vi "Main_17B.vi"() -> ()   [LabVIEW 2024]
uses:
  MAP_Registers.ctl
  ENUM_Instructions.ctl
  <vilib>/Utility/error.llb/Trim Whitespace One-Sided.vi
  Utility/Universal Utility/TypeDefs_Utility/Cluster_Row-Column.ctl
  ENUM_Combo Select.ctl
panel:
  out "Program itteration":i32
  out "A Itteration":i32
  out "Answer":i32
  out "Register start":T1
  out "Output":i32[](array[numeric])
  out "Register end":T1
  in  "Select Data":enum32{"Example", "Puzzle"}(tab)
  in  "Example":string="Register A: 2024\nRegister B: 0\nRegister C: 0\n\nProgram: 0,3,5,4,3,0"
  in  "Puzzle":string="Register A: 60589763\nRegister B: 0\nRegister C: 0\n\nProgram: 2,4,1,5,7,5,1,6,4,1,5,5,0,3,3,0"
  out "Program":i32[](array[numeric])
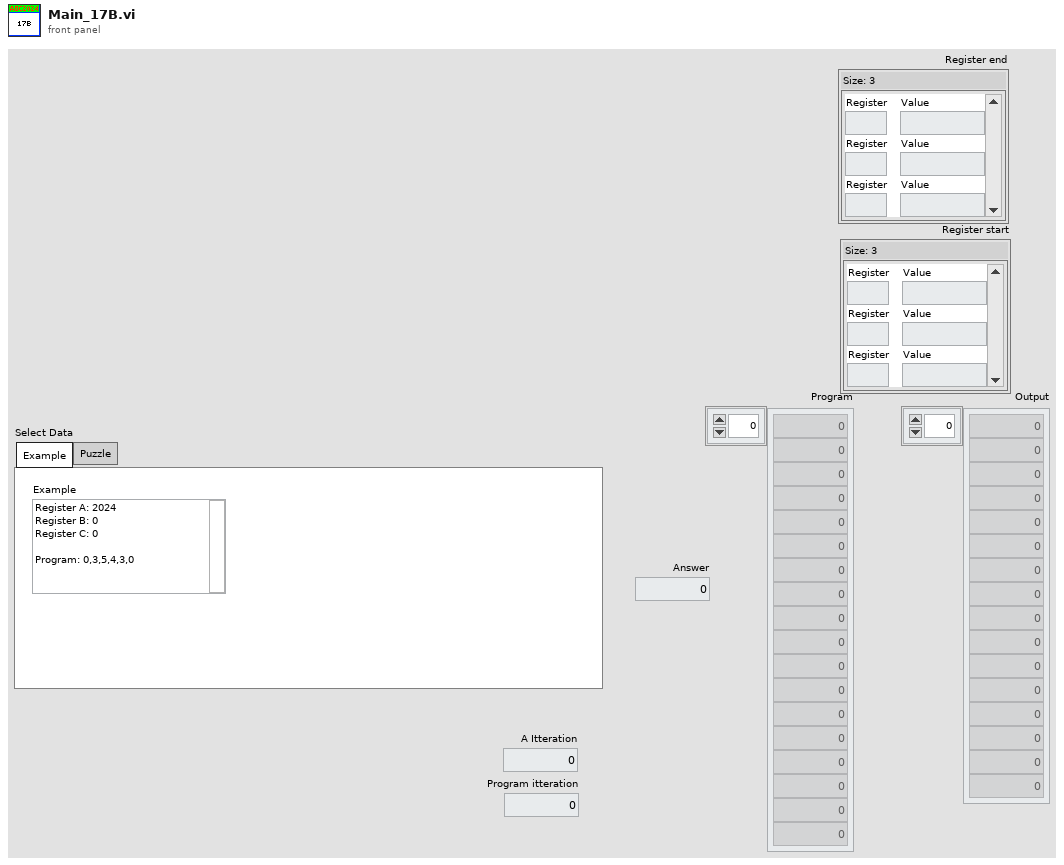
[diagram p1: front panel]
types:
  T1 = typedef "MAP_Registers.ctl" = map{string, i32}
  T2 = typedef "ENUM_Instructions.ctl" = enum16{"adv: [A/(2^combo)] Truncated TO A", "bxl: [B XOR literal] TO B", "bst: [combo MOD 8] TO B", "jnz: [jump Pointer litteral]", "bxc: [B XOR C] TO B", "out: [combo MOD 8] TO OUT", "bdv: [A/(2^combo)] Truncated TO B", "cdv:  [A/(2^combo)] Truncated TO C"}
  T3 = typedef "ENUM_Combo Select.ctl" = enum16{"0", "1", "2", "3", "A", "B", "C", "XXX"}
  T4 = typedef "Cluster_Row-Column.ctl" = cluster{"R":i32, "C":i32}
  T5 = typedef "ENUM_Instructions.ctl" = enum16{"adv: 0 [A/(2^combo)] Truncated TO A", "bxl: 1 [B XOR literal] TO B", "bst: 2 [combo MOD 8] TO B", "jnz: 3 [jump Pointer litteral]", "bxc: 4 [B XOR C] TO B", "out: 5 [combo MOD 8] TO OUT", "bdv: 6 [A/(2^combo)] Truncated TO B", "cdv: 7 [A/(2^combo)] Truncated TO C"}
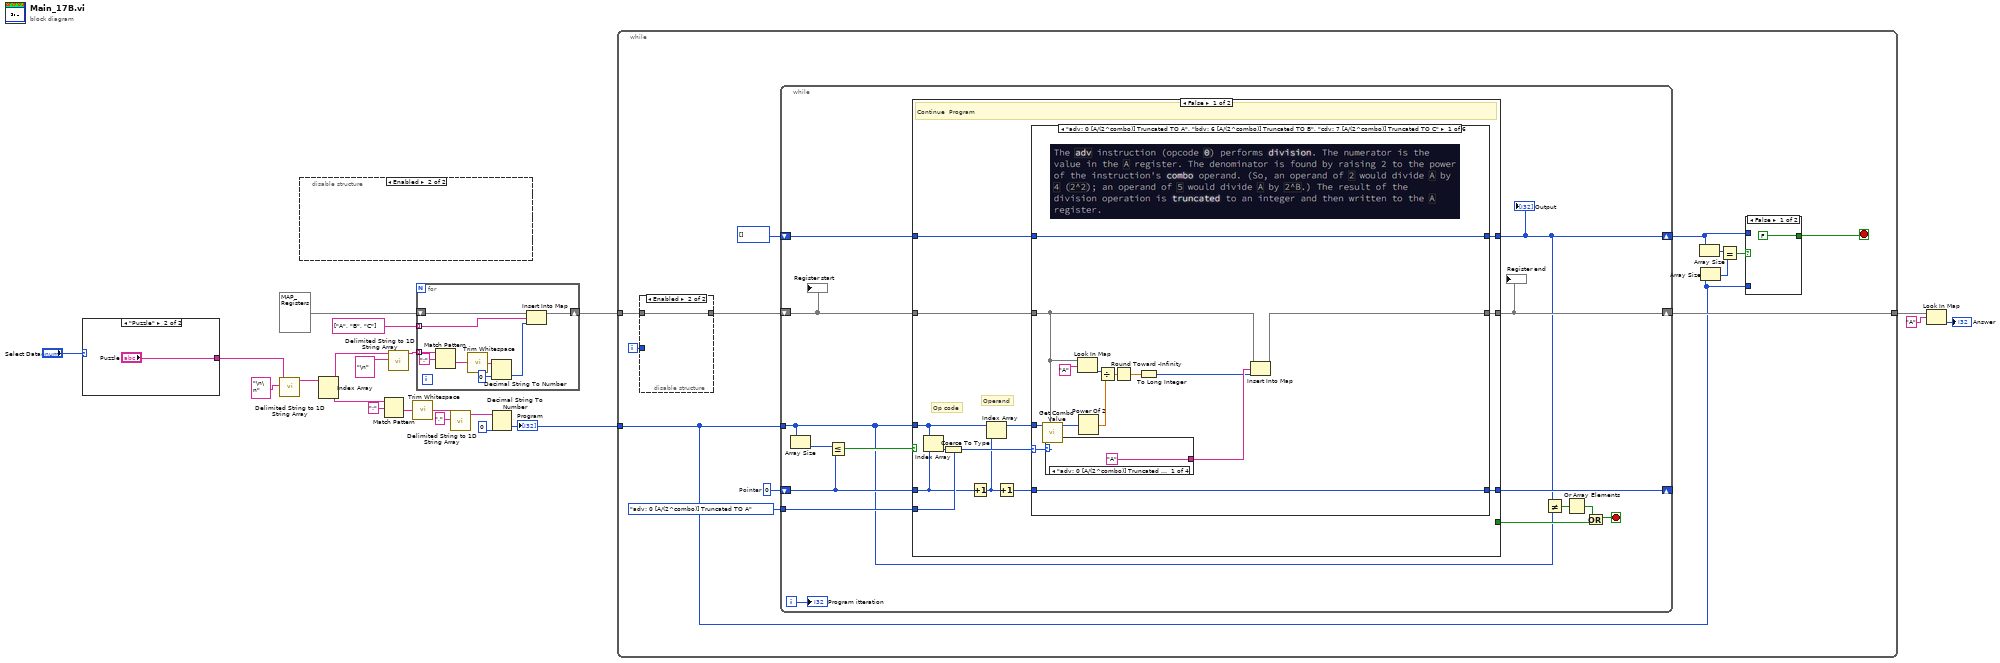
[diagram p0: block diagram]
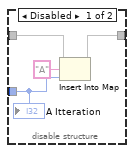
[diagram p2: hidden frame]
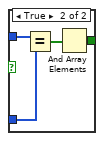
[diagram p3: hidden frame]
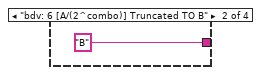
[diagram p4: hidden frame]
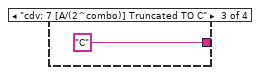
[diagram p5: hidden frame]
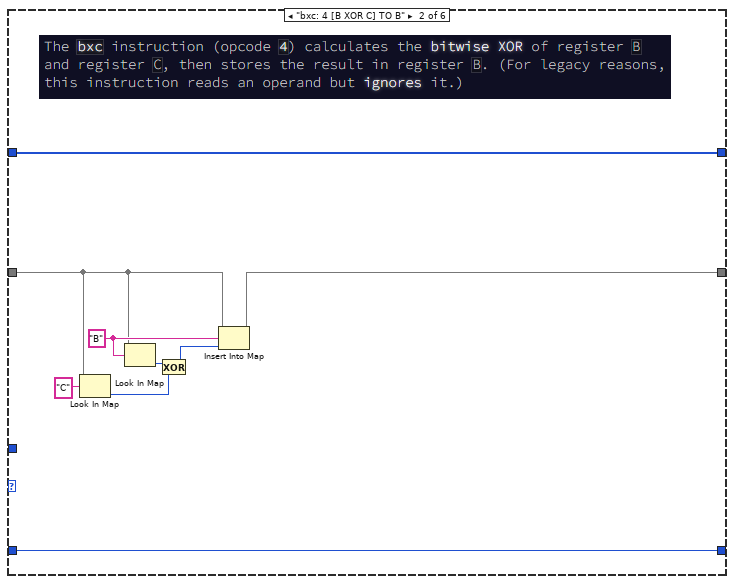
[diagram p7: hidden frame]
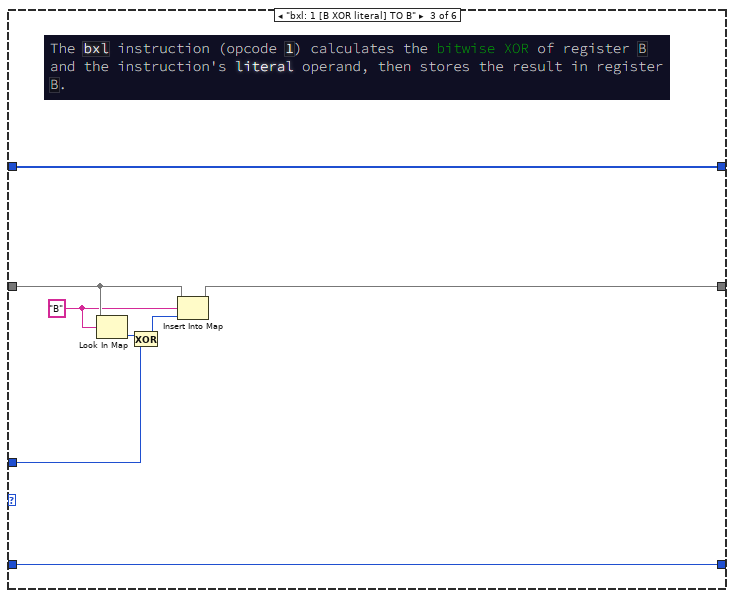
[diagram p8: hidden frame]
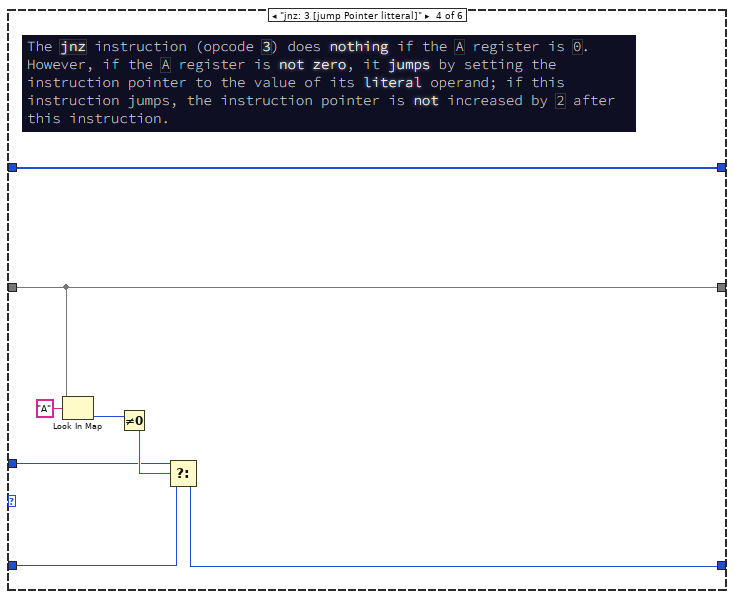
[diagram p9: hidden frame]
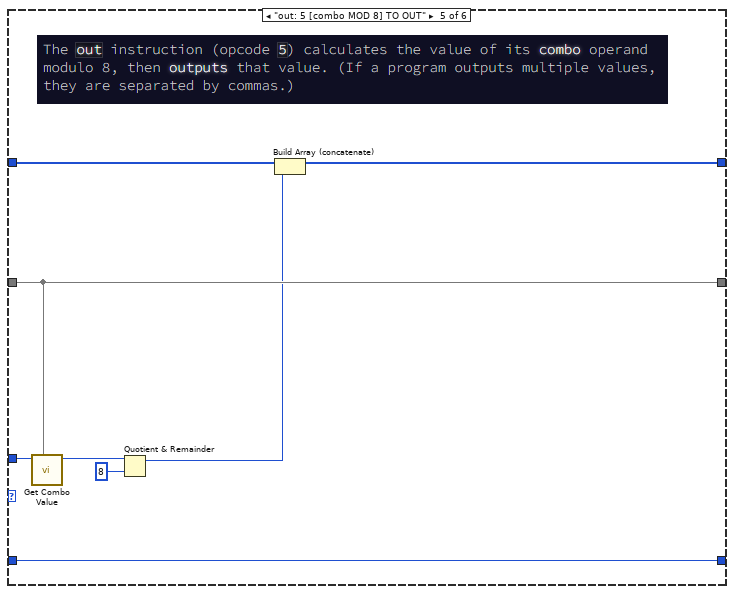
[diagram p10: hidden frame]
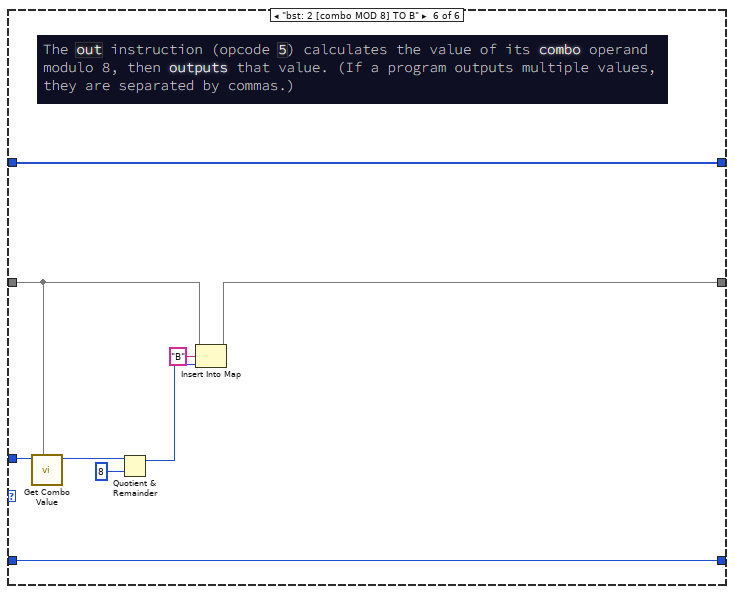
[diagram p11: hidden frame]
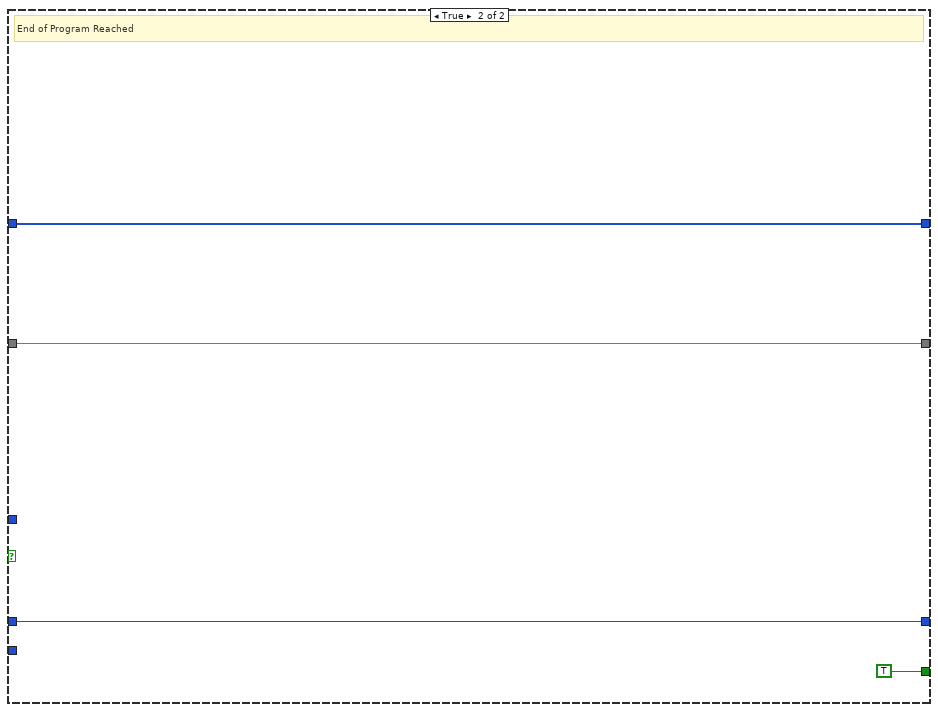
[diagram p12: hidden frame]
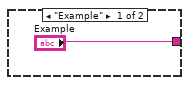
[diagram p13: hidden frame]
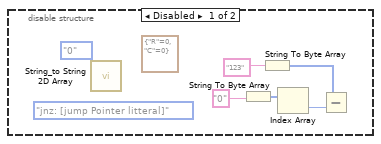
[diagram p14: hidden frame]
diagram:
  n1 = case shown="\"Puzzle\"" "Select Data" {
    tunnel: ["Example" "Puzzle"] -> w4
    frame "Example" {
    }
    frame "Puzzle" {
    }
  }
  n2 = call <vilib>:"Delimited String to 1D String Array.vi"("delimiter"="\n\n" ("delimiter (Tab)"), "delimited string"=w4) -> ("string array"=w20:string[])  [unwired: 9 in]
  n3 = disable-structure shown="Enabled" {
    frame Disabled {
      (unwired) ENUM_Instructions."jnz: [jump Pointer litteral]" ("Instructions")
      (unwired) ENUM_Combo_Select."0" ("Combo")
      (unwired) T4 {"R"=0, "C"=0} ("Position")
      n4 = call "String_to String 2D Array.vi"() -> ()  [unwired: 11 in, 1 out]
      n5 = String To Byte Array(string="0") -> (unsigned byte array=w26:u8[])
      n6 = String To Byte Array(string="123") -> (unsigned byte array=w24:u8[])
      n7 = Index Array(array=w26) -> (element=w25:u8)  [unwired: 1 in]
      n8 = Subtract(x=w24, y=w25) -> ()  [unwired: 1 out]
    }
    frame Enabled {
    }
  }
  n9 = Index Array(array=w20) -> (element #1=w19:string, element #2=w14:string)  [unwired: 2 in]
  n10 = Match Pattern(string=w14, regular expression=":") -> (after substring=w12:string)  [unwired: 1 in, 3 out]
  n11 = call <vilib>:"Delimited String to 1D String Array.vi"("delimiter"="\n" ("delimiter (Tab)"), "delimited string"=w19) -> ("string array"=w17:string[])  [unwired: 9 in]
  n12 = call <vilib>:"Trim Whitespace.vi"("string"=w12) -> ("trimmed string"=w11:string)  [unwired: 1 in]
  n13 = for {
    tunnel: w17 -> [w37] mode=indexing
    shift-right: [w32] -> w7
    shift-left: T1 {} -> [w33]
    tunnel: string[] ["A", "B", "C"] ("String") -> [w31] mode=indexing
    n14 = Match Pattern(string=w37, regular expression=":") -> (after substring=w35:string)  [unwired: 1 in, 3 out]
    n15 = call <vilib>:"Trim Whitespace.vi"("string"=w35) -> ("trimmed string"=w34:string)  [unwired: 1 in]
    n16 = Decimal String To Number(string=w34, default (0L)=u64 0 ("default (0 I32)")) -> (number=w30:u64)  [unwired: 1 in, 1 out]
    n17 = Insert Into Map(map in=w33, key=w31, value=w30) -> (map out=w32:T1)  [unwired: 2 out]
  }
  n18 = call <vilib>:"Delimited String to 1D String Array.vi"("delimiter"=",", "delimited string"=w11) -> ("string array"=w9:string[])  [unwired: 9 in]
  n19 = Decimal String To Number(string=w9, default (0L)=0 ("default (0 I32)")) -> (number=w6:i32[])  [unwired: 1 in, 1 out]
  "Program" <- w6
  n20 = while {
    tunnel: w7 -> [w44]
    tunnel: [w47] -> w3
    tunnel: w6 -> [w39]
    i -> [w46]
    stop <- w38 stop-if-true
    w50 = 0  # Pointer
    n21 = disable-structure shown="Enabled" {
      disable-tunnel: w46 -> [w54 _]
      disable-tunnel: [w52 w55] -> w45
      disable-tunnel: w44 -> [w51 w55]
      frame Disabled {
        n22 = Insert Into Map(map in=w51, key="A", value=w54) -> (map out=w52:T1)  [unwired: 2 out]
        "A Itteration" <- w54
      }
      frame Enabled {
      }
    }
    n23 = while {
      shift-right: [w68] -> w47
      shift-left: w45 -> [w67]
      tunnel: w39 -> [w62]
      shift-right: [w71] -> _
      shift-left: w50 -> [w75]
      shift-right: [w65] -> w40
      shift-left: i32[] [] -> [w73]
      tunnel: ENUM_Instructions."adv: 0 [A/(2^combo)] Truncated TO A" ("Instructions") -> [w72]
      i -> [w61]
      stop <- w66 stop-if-true
      n24 = Array Size(array=w62) -> (size(s)=w69:i32)
      n25 = Less Or Equal?(x=w69, y=w75) -> (x <= y?=w74:bool)
      n26 = case shown="False" w74 {
        tunnel: w62 -> [w78 _]
        tunnel: w75 -> [w81 w150]
        tunnel: w67 -> [w83 w149]
        tunnel: w73 -> [w85 w151]
        tunnel: w72 -> [w86 _]
        tunnel: [w84 w151] -> w65
        tunnel: [w76 w150] -> w71
        tunnel: [w82 w149] -> w68
        tunnel: [_ TRUE] -> w70
        frame False {
          # "Operand"
          # "Op code"
          # "Continue  Program"
          n27 = Index Array(array=w78, index=w81) -> (element=w88:i32)
          n28 = Coerce To Type(0:w88, 1:w86) -> (2:w87:T5)
          n29 = Increment(x=w81) -> (x+1=w80:i32)
          n30 = Index Array(array=w78, index=w80) -> (element=w79:i32)
          n31 = Increment(x=w80) -> (x+1=w77:i32)
          n32 = case shown="\"adv: 0 [A/(2^combo)] Truncated TO A\", \"bdv: 6 [A/(2^combo)] Truncated TO B\", \"cdv: 7 [A/(2^combo)] Truncated TO C\"" w87 {
            selector: w87 -> [w93 _ _ _ _ _]
            tunnel: w79 -> [w100 _ w115 w125 w136 w145]
            tunnel: w85 -> [w102 w114 w122 w130 w138 w147]
            tunnel: [w102 w114 w122 w130 w132 w147] -> w84
            tunnel: w83 -> [w91 w108 w119 w129 w135 w141]
            tunnel: [w92 w112 w120 w129 w135 w142] -> w82
            tunnel: w77 -> [w101 w113 w121 w123 w137 w146]
            tunnel: [w101 w113 w121 w124 w137 w146] -> w76
            frame "adv: 0 [A/(2^combo)] Truncated TO A", "bdv: 6 [A/(2^combo)] Truncated TO B", "cdv: 7 [A/(2^combo)] Truncated TO C" {
              n33 = call "Get Combo Value.vi"("Register Map"=w91, "Operand"=w100) -> ("Combo Value"=w99:i32)  [unwired: 9 in]
              n34 = case shown="\"adv: 0 [A/(2^combo)] Truncated TO A\"" w93 {
                tunnel: ["A" ("key") "B" ("key") "C" ("key") _] -> w90
                frame "adv: 0 [A/(2^combo)] Truncated TO A" {
                }
                frame "bdv: 6 [A/(2^combo)] Truncated TO B" {
                }
                frame "cdv: 7 [A/(2^combo)] Truncated TO C" {
                }
                frame Default {
                }
              }
              n35 = Look In Map(map=w91, key="A") -> (value=w96:i32)  [unwired: 1 in, 1 out]
              n36 = Power Of 2(x=w99) -> (2^x=w97:dbl)
              n37 = Divide(x=w96, y=w97) -> (x/y=w95:dbl)
              n38 = Round Toward -Infinity(1:w95) -> (0:w94:dbl)
              n39 = To Long Integer(number=w94) -> (32bit integer=w89:i32)
              n40 = Insert Into Map(map in=w91, key=w90, value=w89) -> (map out=w92:T1)  [unwired: 2 out]
            }
            frame "bxc: 4 [B XOR C] TO B" {
              w111 = "B" ("key")
              n41 = Look In Map(map=w108, key="C") -> (value=w106:i32)  [unwired: 1 in, 1 out]
              n42 = Look In Map(map=w108, key=w111) -> (value=w110:i32)  [unwired: 1 in, 1 out]
              n43 = Exclusive Or(1:w106, 2:w110) -> (0:w109:i32)
              n44 = Insert Into Map(map in=w108, key=w111, value=w109) -> (map out=w112:T1)  [unwired: 2 out]
            }
            frame "bxl: 1 [B XOR literal] TO B" {
              w118 = "B" ("key")
              n45 = Look In Map(map=w119, key=w118) -> (value=w117:i32)  [unwired: 1 in, 1 out]
              n46 = Exclusive Or(1:w115, 2:w117) -> (0:w116:i32)
              n47 = Insert Into Map(map in=w119, key=w118, value=w116) -> (map out=w120:T1)  [unwired: 2 out]
            }
            frame "jnz: 3 [jump Pointer litteral]" {
              n48 = Look In Map(map=w129, key="A") -> (value=w127:i32)  [unwired: 1 in, 1 out]
              n49 = Not Equal To 0?(x=w127) -> (x != 0?=w126:bool)
              n50 = Select(t=w125, s=w126, f=w123) -> (s? t:f=w124:i32)
            }
            frame "out: 5 [combo MOD 8] TO OUT" {
              n51 = call "Get Combo Value.vi"("Register Map"=w135, "Operand"=w136) -> ("Combo Value"=w134:i32)  [unwired: 9 in]
              n52 = Quotient & Remainder(x=w134, y=8) -> (x-y*floor(x/y)=w131:i32)  [unwired: 1 out]
              n53 = Build Array (concatenate)(w138, w131) -> (w132:i32[])
            }
            frame "bst: 2 [combo MOD 8] TO B" {
              n54 = call "Get Combo Value.vi"("Register Map"=w141, "Operand"=w145) -> ("Combo Value"=w144:i32)  [unwired: 9 in]
              n55 = Quotient & Remainder(x=w144, y=8) -> (x-y*floor(x/y)=w139:i32)  [unwired: 1 out]
              n56 = Insert Into Map(map in=w141, key="B", value=w139) -> (map out=w142:T1)  [unwired: 2 out]
            }
          }
        }
        frame True {
          # "End of Program Reached"
        }
      }
      "Register end" <- w68
      "Output" <- w65
      n57 = Not Equal?(x=w65, y=w62) -> (x != y?=w64:bool[])
      n58 = Or Array Elements(Boolean array=w64) -> (logical OR=w63:bool)
      n59 = Or(x=w63, y=w70) -> (x .or. y?=w66:bool)
      "Register start" <- w67
      "Program itteration" <- w61
    }
    n60 = Array Size(array=w40) -> (size(s)=w42:i32)
    n61 = Array Size(array=w39) -> (size(s)=w43:i32)
    n62 = Equal?(x=w42, y=w43) -> (x = y?=w41:bool)
    n63 = case shown="False" w41 {
      tunnel: w39 -> [_ w60]
      tunnel: w40 -> [_ w59]
      tunnel: [FALSE w57] -> w38
      frame False {
      }
      frame True {
        n64 = Equal?(x=w59, y=w60) -> (x = y?=w58:bool[])
        n65 = And Array Elements(Boolean array=w58) -> (logical AND=w57:bool)
      }
    }
  }
  n66 = Look In Map(map=w3, key="A") -> (value=→"Answer":i32)  [unwired: 1 in, 1 out]
